vi "Configure Marker Peak Search.vi"(0 "VISA resource name":refnum<visa-resource-name>, 1 "Enable Peak Excursion (T: Enable)":bool=TRUE, 2 "Enable Peak Threshold (T: Enable)":bool=TRUE, 3 "Enable Continuous Peak Search (F: Disable)":bool, 5 "Active Marker (1: Marker1)":i32(ring)=1 items=["Marker1"=1, "Marker2"=2, "Marker3"=3, "Marker4"=4, "Marker5"=5, "Marker6"=6, "Marker7"=7, "Marker8"=8, "Marker9"=9, "Marker10"=10, "Marker11"=11, "Marker12"=12], 7 "Marker Search (0: Highest)":i32(ring) items=["Highest", "Next Peak", "Next Peak Left", "Next Peak Right", "Pk-Pk Search", "Minimum"], 9 "Peak Search Criteria (0: Highest Peak)":i32(ring) items=["Highest Peak", "Same as \"Next Peak\" Criteria"], 11 "error in (no error)":errorcluster, 12 "Peak Excursion (6 dB)":dbl=6.0, 13 "Peak Threshold (-90 dBm)":dbl=-90.0) -> (4 "VISA resource name out":refnum<visa-resource-name>, 15 "error out":errorcluster)   [LabVIEW 2018, in "Agilent MXA Series.lvlib"]
doc: "Places the selected marker on the highest signal peak.\n\n<B>Note:</B>\nYou can use this VI only under Swept SA, ACP, Spurious Emissions measurement types."
uses:
  Agilent MXA Series.lvlib
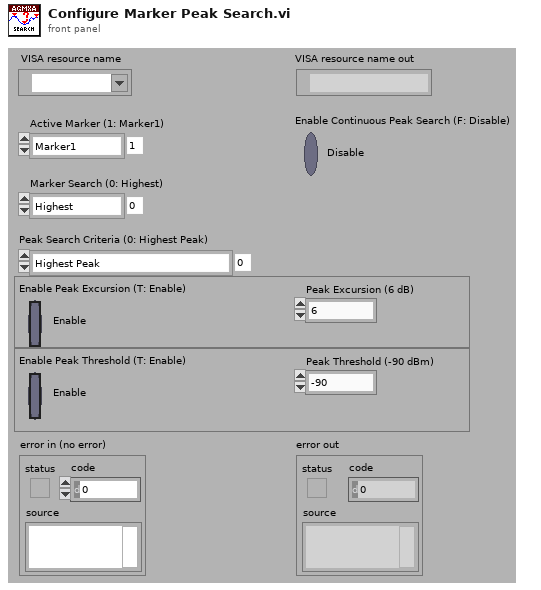
[diagram p1: front panel]
types:
  T1 = typedef "Agilent MXA Series.lvlib/Extended User Data.ctl" = cluster{"Measurement Type":i32, "Agilent MXA/EXA Model":i32}
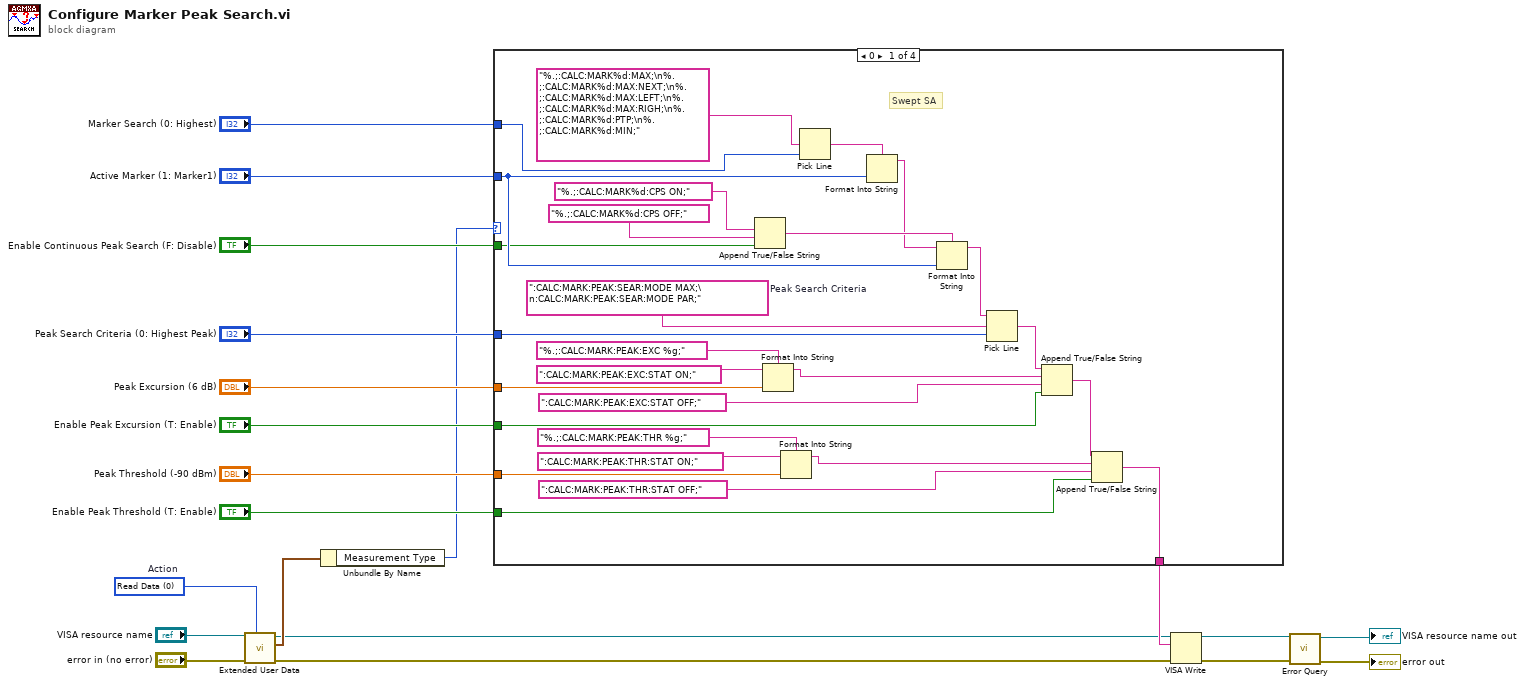
[diagram p0: block diagram]
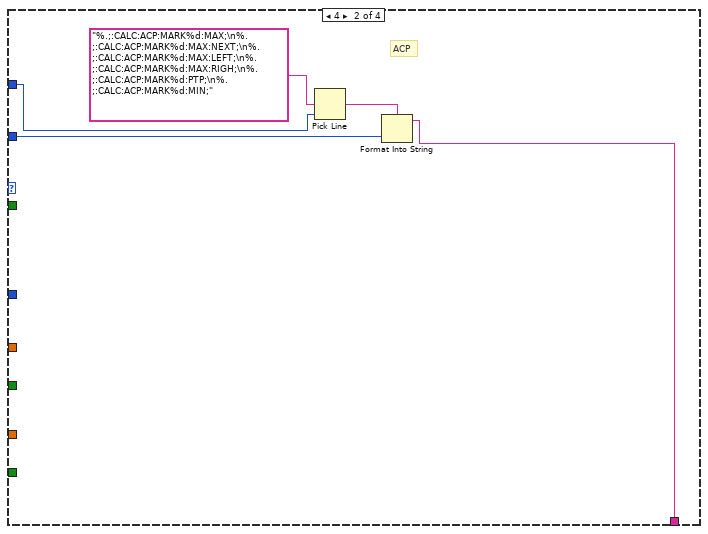
[diagram p2: hidden frame]
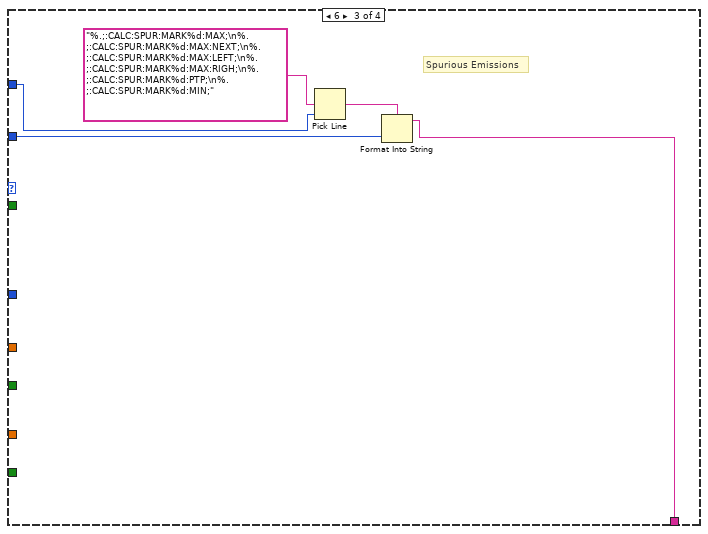
[diagram p3: hidden frame]
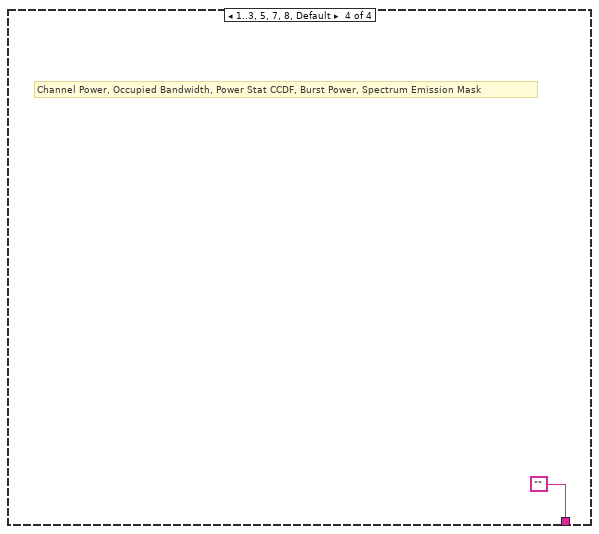
[diagram p4: hidden frame]
diagram:
  w1 = 0 items=["Read Data", "Write Data", "Clear Data", "Clear ALL Data"]  # Action
  n1 = call "Extended User Data.vi"("Action (1:Write Data)"=w1, "Error In (no error)"="error in (no error)", "VISA resource name in"="VISA resource name") -> ("Error Out"=w2:errorcluster, "User Data Out"=w10:T1, "VISA resource name out"=w3:refnum<visa-resource-name>)  [unwired: 6 in]
  n2 = Unbundle By Name(w10) -> ("Measurement Type"=w9:i32)
  n3 = case shown="0" w9 {
    tunnel: "Active Marker (1: Marker1)" -> [w44 w49 w54 _]
    tunnel: "Marker Search (0: Highest)" -> [w46 w51 w56 _]
    tunnel: "Enable Continuous Peak Search (F: Disable)" -> [w41 _ _ _]
    tunnel: "Peak Search Criteria (0: Highest Peak)" -> [w40 _ _ _]
    tunnel: "Peak Excursion (6 dB)" -> [w38 _ _ _]
    tunnel: "Enable Peak Excursion (T: Enable)" -> [w32 _ _ _]
    tunnel: "Peak Threshold (-90 dBm)" -> [w27 _ _ _]
    tunnel: "Enable Peak Threshold (T: Enable)" -> [w26 _ _ _]
    tunnel: [w24 w48 w53 ""] -> w8
    frame 0 {
      w39 = ":CALC:MARK:PEAK:SEAR:MODE MAX;\n:CALC:MARK:PEAK:SEAR:MODE PAR;"  # Peak Search Criteria
      # "Swept SA"
      n4 = Append True/False String(1:w41, 2:"%.;:CALC:MARK%d:CPS OFF;" ("false string"), 3:"%.;:CALC:MARK%d:CPS ON;" ("true string")) -> (0:w23:string)  [unwired: 1 in]
      n5 = Format Into String(format string="%.;:CALC:MARK:PEAK:EXC %g;", initial string=":CALC:MARK:PEAK:EXC:STAT ON;", w38) -> (resulting string=w35:string)  [unwired: 1 in, 1 out]
      n6 = Format Into String(format string="%.;:CALC:MARK:PEAK:THR %g;", initial string=":CALC:MARK:PEAK:THR:STAT ON;", w27) -> (resulting string=w29:string)  [unwired: 1 in, 1 out]
      n7 = Pick Line(multi-line string="%.;:CALC:MARK%d:MAX;\n%.;:CALC:MARK%d:MAX:NEXT;\n%.;:CALC:MARK%d:MAX:LEFT;\n%.;:CALC:MARK%d:MAX:RIGH;\n%.;:CALC:MARK%d:PTP;\n%.;:CALC:MARK%d:MIN;", line index=w46) -> (output string=w45:string)  [unwired: 1 in]
      n8 = Format Into String(format string=w45, w44) -> (resulting string=w22:string)  [unwired: 2 in, 1 out]
      n9 = Format Into String(format string=w23, initial string=w22, w44) -> (resulting string=w21:string)  [unwired: 1 in, 1 out]
      n10 = Pick Line(string ("")=w21, multi-line string=w39, line index=w40) -> (output string=w34:string)
      n11 = Append True/False String(1:w32, 2:":CALC:MARK:PEAK:EXC:STAT OFF;" ("false string"), 3:w35, 4:w34) -> (0:w25:string)
      n12 = Append True/False String(1:w26, 2:":CALC:MARK:PEAK:THR:STAT OFF;" ("false string"), 3:w29, 4:w25) -> (0:w24:string)
    }
    frame 4 {
      # "ACP"
      n13 = Pick Line(multi-line string="%.;:CALC:ACP:MARK%d:MAX;\n%.;:CALC:ACP:MARK%d:MAX:NEXT;\n%.;:CALC:ACP:MARK%d:MAX:LEFT;\n%.;:CALC:ACP:MARK%d:MAX:RIGH;\n%.;:CALC:ACP:MARK%d:PTP;\n%.;:CALC:ACP:MARK%d:MIN;", line index=w51) -> (output string=w50:string)  [unwired: 1 in]
      n14 = Format Into String(format string=w50, w49) -> (resulting string=w48:string)  [unwired: 2 in, 1 out]
    }
    frame 6 {
      # "Spurious Emissions"
      n15 = Pick Line(multi-line string="%.;:CALC:SPUR:MARK%d:MAX;\n%.;:CALC:SPUR:MARK%d:MAX:NEXT;\n%.;:CALC:SPUR:MARK%d:MAX:LEFT;\n%.;:CALC:SPUR:MARK%d:MAX:RIGH;\n%.;:CALC:SPUR:MARK%d:PTP;\n%.;:CALC:SPUR:MARK%d:MIN;", line index=w56) -> (output string=w55:string)  [unwired: 1 in]
      n16 = Format Into String(format string=w55, w54) -> (resulting string=w53:string)  [unwired: 2 in, 1 out]
    }
    frame 1..3, 5, 7, 8, Default {
      # "Channel Power, Occupied Bandwidth, Power Stat CCDF, Burst Power, Spectrum Emission Mask"
    }
  }
  n17 = VISA Write(VISA resource name=w3, write buffer=w8, error in (no error)=w2) -> (VISA resource name out=w7:refnum<visa-resource-name>, error out=w6:errorcluster)  [unwired: 1 out]
  n18 = call "Error Query.vi"("error in (no error)"=w6, "VISA resource name"=w7) -> ("error out"=→"error out":errorcluster, "VISA resource name out"=→"VISA resource name out":refnum<visa-resource-name>)  [unwired: 6 in, 2 out]
